vi "Actor Core.vi"(8 "error in":errorcluster, 11 "Measure Object in":refnum<class "Error Log.lvclass">) -> (0 "error out":errorcluster, 3 "Actor out":refnum<class "Actor.lvclass">)   [LabVIEW 2024, in "Error Log.lvclass"]
doc: "(<B>Filename</B>: Actor Framework.lvlib:Actor.lvclass:Actor Core.vi)\n\nReceives messages to the actor, reacts to them, and initiates any error handling that may shut the actor down.\n\nDescendant classes may override this VI to append parallel tasks for the actor to complete while it handles messages. Overrides use the Call Parent Method node."
uses:
  Error Log.lvclass
  <vilib>/ActorFramework/Actor/Actor.lvclass
  Worker/Worker Actor/Worker Actor.lvclass
panel:
  out "Log file":string
  out "Error log":string
  out "Name":string
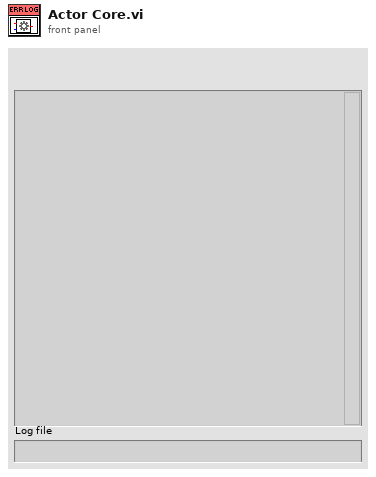
[diagram p1: front panel]
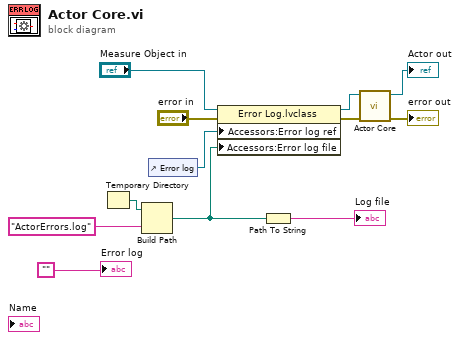
[diagram p0: block diagram]
diagram:
  n1 = Temporary Directory() -> (w4:path)
  n2 = Build Path(base path=w4, name or relative path="ActorErrors.log") -> (appended path=w2:path)
  n3 = control-ref of="Error log"() -> (w6:refnum<vi>)
  n4 = property class="Error Log.lvclass"(reference="Measure Object in", error in="error in", "Accessors:Error log ref"=w6, "Accessors:Error log file"=w2) -> (reference out=w7:refnum<class "Error Log.lvclass">, error out=w9:errorcluster)
  n5 = Path To String(path=w2) -> (string=→"Log file":string)
  n6 = call-parent "Actor Core.vi"("error in"=w9, "Measure Object in"=w7) -> ("error out"=→"error out":errorcluster, "Actor out"=→"Actor out":refnum<class "Actor.lvclass">)  [unwired: 8 in]
  "Error log" <- ""
